vi "__sanatizeURL.vi"(11 "url in":string) -> (3 "url out":string)   [LabVIEW 2020, in "REST_Client.lvclass"]
uses:
  REST_Client.lvclass
  <vilib>/Utility/error.llb/whitespace.ctl
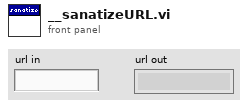
[diagram p1: front panel]
types:
  T1 = typedef "whitespace.ctl" = u16
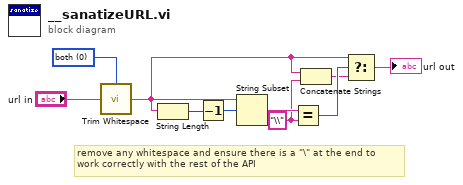
[diagram p0: block diagram]
diagram:
  w3 = "\\"
  w9 = T1 0 items=["both", "start of string", "end of string"] ("location (both)")
  # "remove any whitespace and ensure there is a \"\\\" at the end to \nwork correctly with the rest of the API"
  n1 = call <vilib>:"Trim Whitespace.vi"("string"="url in", "location (both)"=w9) -> ("trimmed string"=w4:string)
  n2 = String Length(string=w4) -> (length=w8:i32)
  n3 = Decrement(x=w8) -> (x-1=w7:i32)
  n4 = String Subset(string=w4, offset (0)=w7) -> (substring=w6:string)  [unwired: 1 in]
  n5 = Equal?(x=w6, y=w3) -> (x = y?=w5:bool)
  n6 = Concatenate Strings(w4, w3) -> (w2:string)
  n7 = Select(t=w4, s=w5, f=w2) -> (s? t:f=→"url out":string)
